vi "Make DLL Param(Storage Info).vi"(1 "Storage Info":T1) -> (0 "pStorageInfo":T2)   [LabVIEW 8.6, in "Keyence LJ-V7000.lvlib"]
uses:
  Keyence LJ-V7000.lvlib
  Public/Clusters/Storage Info.ctl
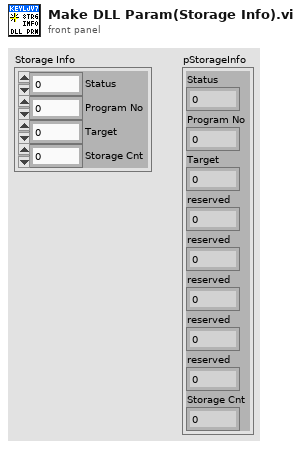
[diagram p1: front panel]
types:
  T1 = typedef "Keyence LJ-V7000.lvlib/Storage Info.ctl" = cluster{"Status":u8, "Program No":u8, "Target":u8, "Storage Cnt":u32}
  T2 = cluster{"Status":u8, "Program No":u8, "Target":u8, "reserved":u8, "reserved":u8, "reserved":u8, "reserved":u8, "reserved":u8, "Storage Cnt":u32}
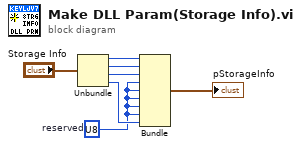
[diagram p0: block diagram]
diagram:
  w5 = u8 ?  # reserved
  n1 = Unbundle("Storage Info") -> ("Status"=w2:u8, "Program No"=w3:u8, "Target"=w4:u8, "Storage Cnt"=w6:u32)
  n2 = Bundle("Status"=w2, "Program No"=w3, "Target"=w4, "reserved"=w5, "reserved"=w5, "reserved"=w5, "reserved"=w5, "reserved"=w5, "Storage Cnt"=w6) -> (→"pStorageInfo":T2)  [unwired: 1 in]
